vi "fastFrame_wave_to_bg_and_mol_signal.vi"(1 "all fast frames":dbl[](array[numeric])) -> (4 "bg frames":dbl[][](array[numeric]), 6 "mol. frames":dbl[][](array[numeric]))   [LabVIEW 2011]
doc: "This VI takes the wavform measured by the OSC and calculates the average signal for both the background as well as the molecular cylce. It also creates the substracted array (i.e. molecular - background signal)"
uses:
  global.vi
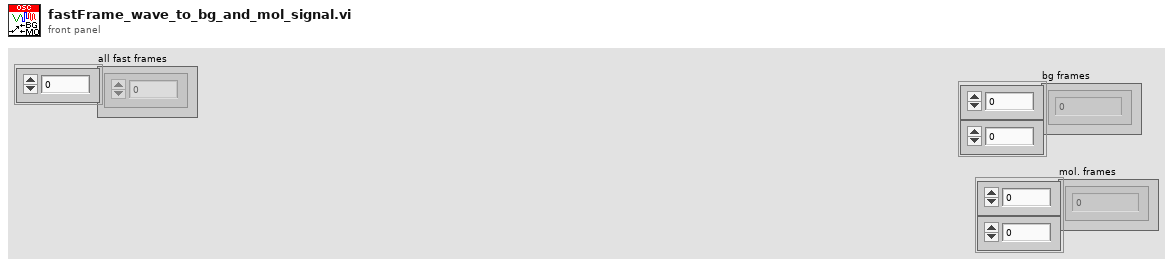
[diagram p1: front panel]
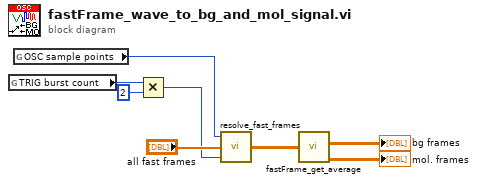
[diagram p0: block diagram]
diagram:
  n1 = global read "global.vi" "TRIG burst count"() -> (w5:i32)
  n2 = global read "global.vi" "OSC sample points"() -> (w7:i32)
  n3 = Multiply(x=w5, y=2) -> (x*y=w3:i32)
  n4 = call "resolve_fast_frames.vi"("fast frame count"=w3, "all fast frames"="all fast frames", "sample points per frame"=w7) -> ("resolved waveforms"=w6:dbl[][])  [unwired: 2 in]
  n5 = call "fastFrame_get_average.vi"("array"=w6) -> ("bg frames"=→"bg frames":dbl[][], "mol. frames"=→"mol. frames":dbl[][])  [unwired: 4 in]
